vi "5T_Queue_Commands.vi"(1 "5T Control":T1 {"Rate (T/min)" format="%6_5f"}, 3 "5T Queue":refnum<queue>) -> (0 "New Status":T1 {"Rate (T/min)" format="%6_5f"})   [LabVIEW 2019]
uses:
  Mischer/5T_Control.ctl
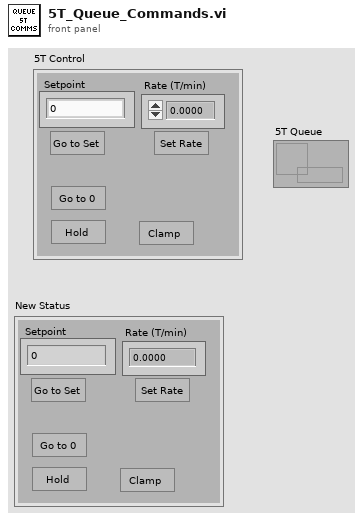
[diagram p1: front panel]
types:
  T1 = typedef "5T_Control.ctl" = cluster{"Rate (T/min)":dbl, "Setpoint":dbl, "Go to set":bool, "Go to Zero":bool, "Clamp":bool, "Go to Hold":bool, "Set Rate":bool}
  T2 = cluster{"Rate (T/min)":bool, "Setpoint":bool, "Go to set":bool, "Go to Zero":bool, "Clamp":bool, "Go to Hold":bool, "Set Rate":bool}
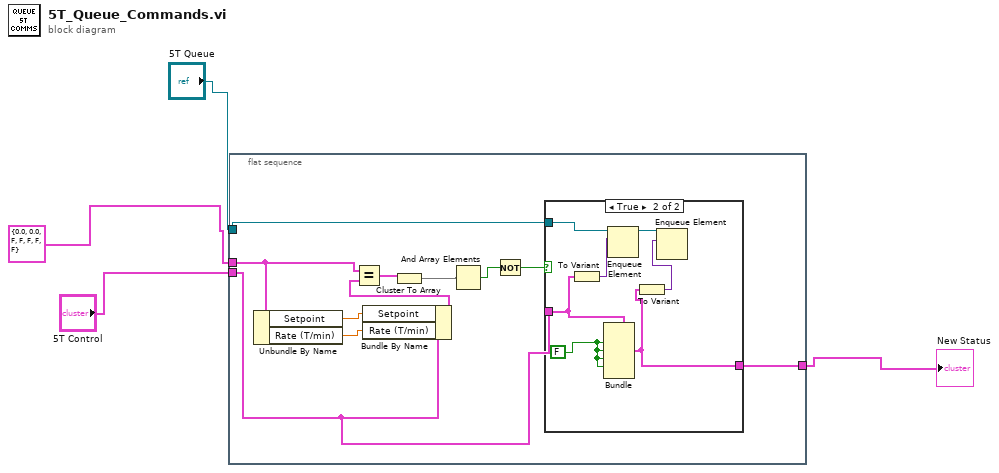
[diagram p0: block diagram]
diagram:
  n1 = flat-sequence {
    tunnel: "5T Queue" -> [w15]
    tunnel: "5T Control" -> [w9]
    tunnel: T1 {"Rate (T/min)"=0.0, "Setpoint"=0.0, "Go to set"=FALSE, "Go to Zero"=FALSE, "Clamp"=FALSE, "Go to Hold"=FALSE, "Set Rate"=FALSE} ("5T Control") -> [w7]
    tunnel: [w10] -> w2
    frame #0 {
      n2 = Unbundle By Name(w7) -> ("Setpoint"=w6:dbl, "Rate (T/min)"=w5:dbl)
      n3 = Bundle By Name(cluster=w9, "Setpoint"=w6, "Rate (T/min)"=w5) -> (w8:T1)
      n4 = Equal?(x=w7, y=w8) -> (x = y?=w11:T2)
      n5 = Cluster To Array(cluster=w11) -> (array=w14:bool[])
      n6 = And Array Elements(Boolean array=w14) -> (logical AND=w13:bool)
      n7 = Not(x=w13) -> (.not. x?=w12:bool)
      n8 = case shown="True" w12 {
        tunnel: w15 -> [_ w23]
        tunnel: w9 -> [w16 w19]
        tunnel: [w16 w18] -> w10
        frame False {
        }
        frame True {
          w17 = FALSE
          n9 = To Variant(anything=w19) -> (Variant=w22:variant)
          n10 = Bundle(cluster=w19, "Go to set"=w17, "Go to Zero"=w17, "Clamp"=w17, "Go to Hold"=w17) -> (w18:T1)  [unwired: 3 in]
          n11 = Enqueue Element(queue=w23, element=w22) -> (queue out=w21:refnum<queue>)  [unwired: 2 in, 2 out]
          n12 = To Variant(anything=w18) -> (Variant=w20:variant)
          n13 = Enqueue Element(queue=w21, element=w20) -> ()  [unwired: 2 in, 3 out]
        }
      }
    }
  }
  "New Status" <- w2
